vi "UDPCupData.vi"(8 "error in (no error)":errorcluster, 11 "UDP Network Connection in":refnum<k16>) -> (0 "error out":errorcluster, 2 "Cup Data":T1, 3 "UDP Network Connection out":refnum<k16>)   [LabVIEW 2017]
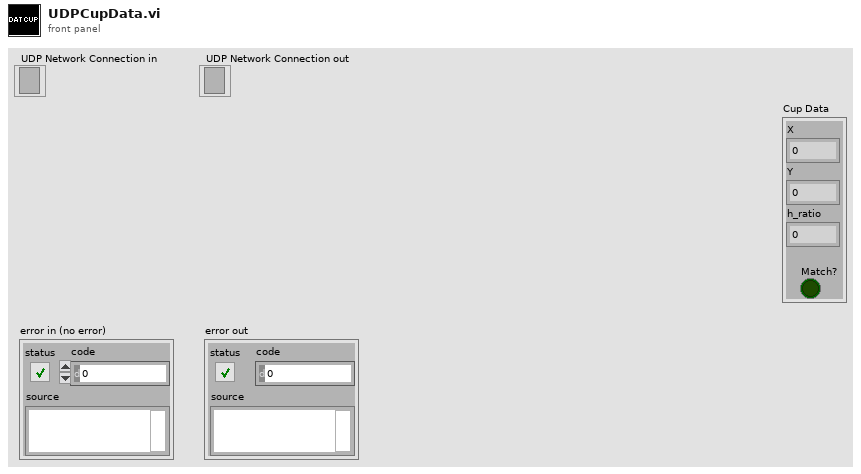
[diagram p1: front panel]
types:
  T1 = cluster{"X":dbl, "Y":dbl, "h_ratio":dbl, "Match?":bool}
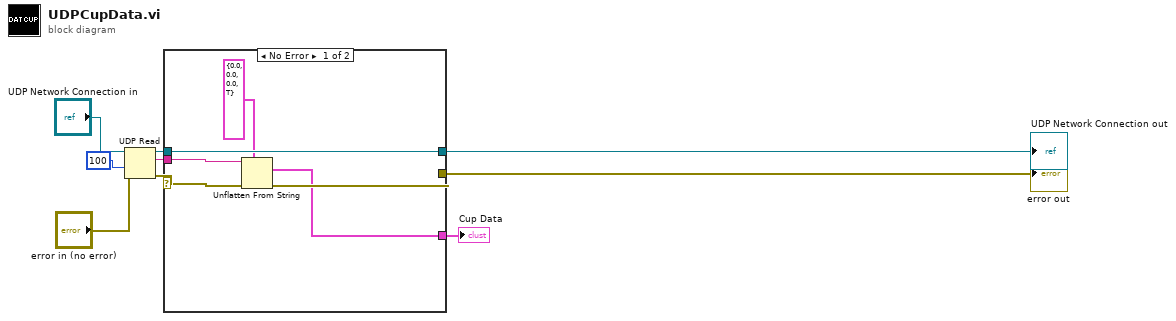
[diagram p0: block diagram]
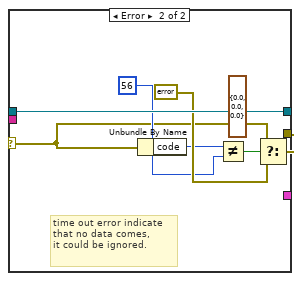
[diagram p2: hidden frame]
diagram:
  n1 = UDP Read(connection ID="UDP Network Connection in", timeout ms (25000)=100, 8:"error in (no error)") -> (data out=w4:string, error out=w6:errorcluster, 3:w8:refnum<k16>)  [unwired: 1 in, 2 out]
  n2 = case shown="No Error" w6 {
    selector: w6 -> [w14 w17]
    tunnel: [w12 w16] -> w7
    tunnel: w4 -> [w15 _]
    tunnel: w8 -> [w13 w22]
    tunnel: [w13 w22] -> w9
    tunnel: [w11 _] -> w1
    frame No Error {
      n3 = Unflatten From String(type=cluster{"X":dbl, "X 2":dbl, "X 3":dbl, bool} {"X"=0.0, "X 2"=0.0, "X 3"=0.0, TRUE}, binary string=w15, error in (no error)=w14) -> (value=w11:cluster{"X":dbl, "X 2":dbl, "X 3":dbl, bool}, error out=w12:errorcluster)  [unwired: 2 in, 1 out]
    }
    frame Error {
      (unwired) cluster{"X":dbl, "Y":dbl, "h_ratio":dbl} {"X"=0.0, "Y"=0.0, "h_ratio"=0.0} ("Cluster")
      # "time out error indicate that no data comes,\nit could be ignored."
      n4 = Unbundle By Name(w17) -> ("code"=w19:i32)
      n5 = Not Equal?(x=w19, y=56) -> (x != y?=w18:bool)
      n6 = Select(t=w17, s=w18, f=errorcluster {"status"=FALSE, "code"=0, "source"=""} ("error out")) -> (s? t:f=w16:errorcluster)
    }
  }
  "UDP Network Connection out" <- w9
  "error out" <- w7
  "Cup Data" <- w1
